vi "Get JSON API Documentation (template).vi"() -> ()   [LabVIEW 2019, in "Help.lvclass"]
uses:
  Help.lvclass
  Help.lvclass/Help.ctl
panel:
  in  "response cluster":variant
  in  "<JSON> response documentation":string
  out "<JSON> API documentation":string
  out "error out":errorcluster
  in  "request cluster":variant
  in  "<JSON> request documentation":string
  in  "command":string
  in  "command description":string
  in  "error in (no error)":errorcluster
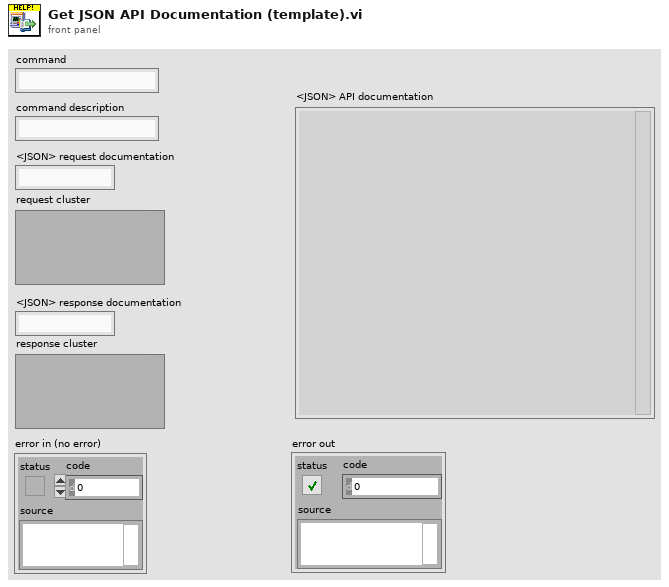
[diagram p1: front panel]
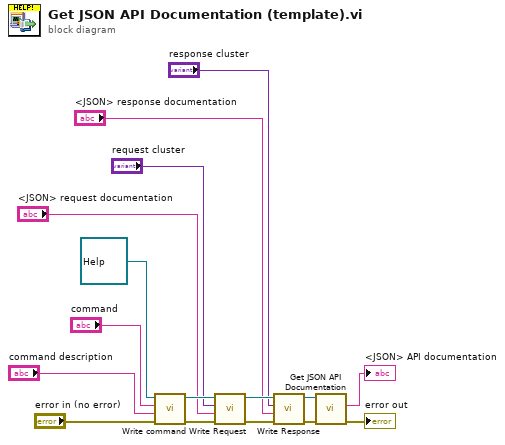
[diagram p0: block diagram]
diagram:
  n1 = call "Write command.vi"("error in (no error)"="error in (no error)", "command description"="command description", "command"="command", "Help in"=refnum<class "Help.lvclass"> refnum) -> ("error out"=w16:errorcluster, "Help out"=w11:refnum<class "Help.lvclass">)  [unwired: 6 in]
  n2 = call "Write Request.vi"("error in (no error)"=w16, "<JSON> request documentation"="<JSON> request documentation", "request cluster"="request cluster", "Help in"=w11) -> ("error out"=w15:errorcluster, "Help out"=w12:refnum<class "Help.lvclass">)  [unwired: 6 in]
  n3 = call "Write Response.vi"("error in (no error)"=w15, "<JSON> response documentation"="<JSON> response documentation", "response cluster"="response cluster", "Help in"=w12) -> ("error out"=w14:errorcluster, "Help out"=w13:refnum<class "Help.lvclass">)  [unwired: 6 in]
  n4 = call "Get JSON API Documentation.vi"("error in (no error)"=w14, "Help"=w13) -> ("error out"=→"error out":errorcluster, "<JSON> API documentation"=→"<JSON> API documentation":string)  [unwired: 7 in, 1 out]
